vi "ManualControlL0NOGENControlled.vi"() -> ()   [LabVIEW 2012]
uses:
  <vilib>/Utility/NIReport.llb/NI_report.lvclass
  <vilib>/Utility/NIReport.llb/HTML/NI_HTML.lvclass
panel:
  in  "Ib Clip select":i32(slide)=63 scale=0.0..63.0
  in  "Clipping Select":i32(slide)=1 scale=1.0..3.0
  in  "Attenuation Select":i32(slide) scale=0.0..15.0
  in  "Channel Enable":i32(slide) scale=0.0..6.0
  in  "Instrument VISA in":T1={"AWG VISA"="AgilentGenerator1", "Oscilloscope  VISA "="AgilentOsciloscope", "Integration Board IP"="172.16.17.47", "connection ID"=refnum, "report out"=refnum, "report file path"=path "C:/Documents and Settings/CTA_LAB01/Desktop/L0_Asic/L0 Asic Test Data"}
  out "error out":errorcluster
  in  "error in":errorcluster
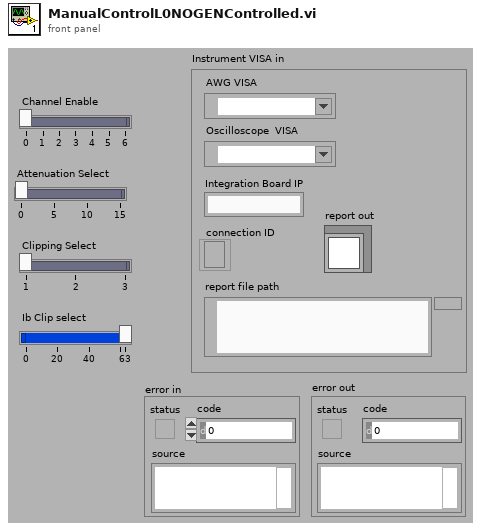
[diagram p1: front panel]
types:
  T1 = cluster{"AWG VISA":refnum<visa-resource-name>, "Oscilloscope  VISA ":refnum<visa-resource-name>, "Integration Board IP":string, "connection ID":refnum<k5>, "report out":refnum<class "NI_report.lvclass">, "report file path":path}
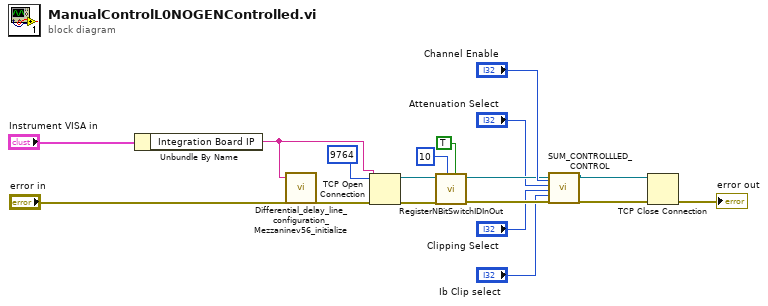
[diagram p0: block diagram]
diagram:
  n1 = Unbundle By Name("Instrument VISA in") -> ("Integration Board IP"=w10:string)
  n2 = call "Differential_delay_line_configuration_Mezzaninev56_initialize.vi"("error in (no error)"="error in", "address"=w10) -> ("error out 2"=w15:errorcluster)  [unwired: 1 in]
  n3 = TCP Open Connection(address=w10, remote port or service name=9764, error in (no error)=w15) -> (connection ID=w13:refnum<k5>, error out=w14:errorcluster)  [unwired: 2 in]
  n4 = call "RegisterNBitSwitchIDInOut.vi"("Switch Bit"=TRUE, "N Bit"=10, "error in (no error)"=w14, "connection ID"=w13) -> ("error out"=w7:errorcluster, "connection ID out"=w4:refnum<k5>)  [unwired: 5 in]
  n5 = call "SUM_CONTROLLLED_CONTROL.vi"("connection ID in"=w4, "Channel Enable"="Channel Enable", "Attenuation Select"="Attenuation Select", "Clipping Select"="Clipping Select", "Ib Clip select"="Ib Clip select", "error in"=w7) -> ("connection ID out"=w5:refnum<k5>, "error out"=w6:errorcluster)  [unwired: 12 in]
  n6 = TCP Close Connection(connection ID=w5, error in (no error)=w6) -> (error out=→"error out":errorcluster)  [unwired: 1 in, 1 out]
